vi "Destroy Buider.vi"(8 "error in (no error)":errorcluster, 11 "CD Build Tools in":refnum<class "Project Build Tools.lvclass">) -> (0 "error out":errorcluster)   [LabVIEW 2019, in "Project Build Tools.lvclass"]
uses:
  Project Build Tools.lvclass
  Project Build Tools.lvclass/Project Build Tools.ctl
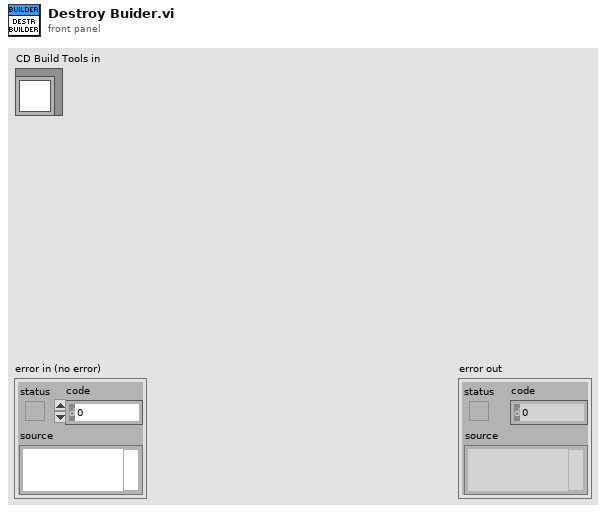
[diagram p1: front panel]
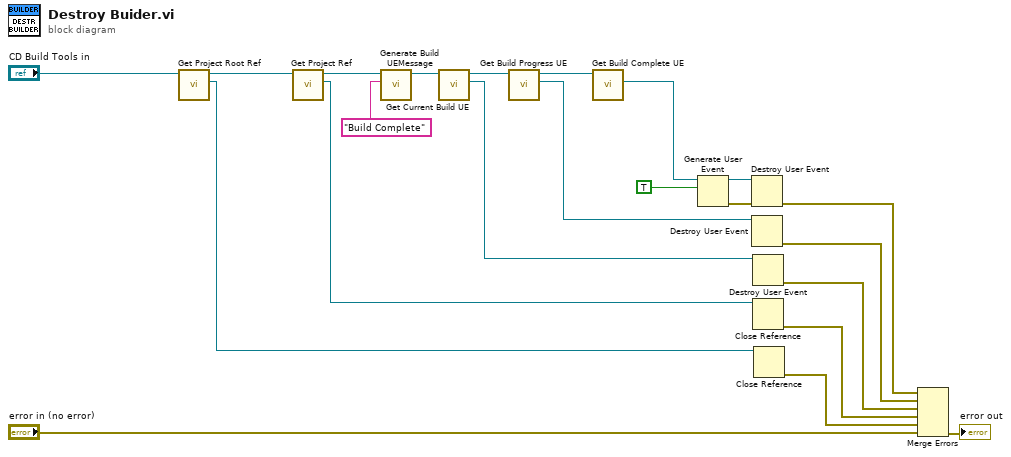
[diagram p0: block diagram]
diagram:
  n1 = call "Get Project Root Ref.vi"("CD Build Tools in"="CD Build Tools in") -> ("Project Root Ref"=w20:refnum<vi>, "CD Build Tools out"=w21:refnum<class "Project Build Tools.lvclass">)  [unwired: 9 in]
  n2 = call "Get Project Ref.vi"("CD Build Tools in"=w21) -> ("Project Ref"=w19:refnum<vi>, "CD Build Tools out"=w3:refnum<class "Project Build Tools.lvclass">)  [unwired: 9 in]
  n3 = call "Generate Build UEMessage.vi"("Message"="Build Complete" ("event data"), "Project Build Tools in"=w3) -> ("Project Build Tools out"=w2:refnum<class "Project Build Tools.lvclass">)  [unwired: 8 in, 1 out]
  n4 = call "Get Current Build UE.vi"("CD Build Tools in"=w2) -> ("Current Build UE"=w4:refnum<user-event>, "CD Build Tools out"=w11:refnum<class "Project Build Tools.lvclass">)  [unwired: 9 in]
  n5 = call "Get Build Progress UE.vi"("CD Build Tools in"=w11) -> ("Build Progress UE"=w14:refnum<user-event>, "CD Build Tools out"=w10:refnum<class "Project Build Tools.lvclass">)  [unwired: 9 in]
  n6 = call "Get Build Complete UE.vi"("CD Build Tools in"=w10) -> ("Build Complete UE"=w9:refnum<user-event>)  [unwired: 9 in, 1 out]
  n7 = Generate User Event(user event=w9, event data cluster=TRUE ("event data")) -> (user event out=w7:refnum<user-event>, error out=w6:errorcluster)  [unwired: 2 in]
  n8 = Destroy User Event(user event=w7, error in=w6) -> (error out=w5:errorcluster)
  n9 = Destroy User Event(user event=w14) -> (error out=w13:errorcluster)  [unwired: 1 in]
  n10 = Destroy User Event(user event=w4) -> (error out=w12:errorcluster)  [unwired: 1 in]
  n11 = Close Reference(reference=w19) -> (error out=w16:errorcluster)  [unwired: 1 in]
  n12 = Close Reference(reference=w20) -> (error out=w17:errorcluster)  [unwired: 1 in]
  n13 = Merge Errors(w5, w13, w12, w16, w17, "error in (no error)") -> (→"error out":errorcluster)
